vi "Pareto CDF.vi"(9 "c":dbl=3.0, 10 "a":dbl=1.0, 11 "x":dbl=4.999999999999998) -> (0 "error":i32, 3 "cdf(x)":dbl=0.992)   [LabVIEW 2014, in "NI_Gmath.lvlib"]
doc: "Computes the continuous cumulative distribution function (CDF), or the probability that the random variate X, where X describes the selected distribution type, has a value less than or equal to <B>x</B>. You must manually select the polymorphic instance to use."
uses:
  NI_Gmath.lvlib
  st_error_code.ctl
panel:
  # "Pareto CDF"
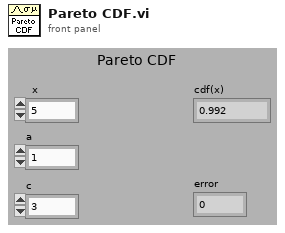
[diagram p1: front panel]
types:
  T1 = typedef "NI_Gmath.lvlib/st_error_code.ctl" = i32
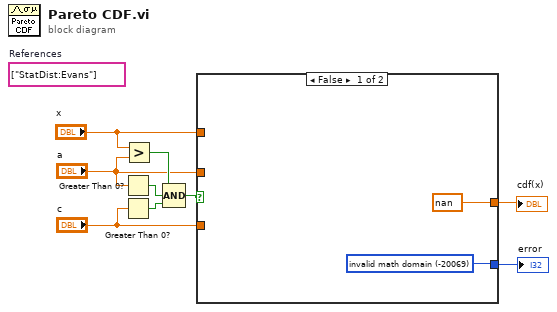
[diagram p0: block diagram]
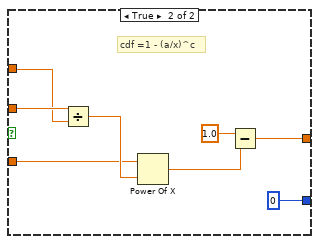
[diagram p2: hidden frame]
diagram:
  (unwired) string[] ["StatDist:Evans"]  # References
  n1 = Greater Than 0?(x="a") -> (x > 0?=w8:bool)
  n2 = Greater Than 0?(x="c") -> (x > 0?=w7:bool)
  n3 = Greater?(x="x", y="a") -> (0:w9:bool)
  n4 = Compound Arithmetic op=AND(w9, w8, w7) -> (w6:bool)
  n5 = case shown="False" w6 {
    tunnel: "c" -> [_ w12]
    tunnel: [w10 0 ("invalid math domain")] -> w4
    tunnel: [nan w16] -> w5
    tunnel: "x" -> [_ w14]
    tunnel: "a" -> [_ w15]
    frame False {
      w10 = T1 -20069 items=["invalid math domain"=-20069, "Fourier interpolation size m >= n"=-20070, "empty array"=-20003] ("stat interp error code")
    }
    frame True {
      # "cdf =1 - (a/x)^c"
      n6 = Divide(x=w15, y=w14) -> (x/y=w13:dbl)
      n7 = Power Of X(1:w13, 2:w12) -> (0:w17:dbl)
      n8 = Subtract(x=1.0, y=w17) -> (x-y=w16:dbl)
    }
  }
  "cdf(x)" <- w5
  "error" <- w4
